vi "Get Label Settings for RT.vi"(8 "error in":errorcluster, 11 "label ref in":T1 format="%.0x") -> (0 "error out":errorcluster, 2 "label settings for RT":T2 {"Label Timestamp Channel Data Reference" format="%.0x"; "Word Initial Raw Value" format="%032.0f"; "Label Disable/Trigger Channel Reference" format="%.0x"; "parameter driver data"."Tx parameter refs" format="%.0x"; "SDI" format="%02b"; "label" format="%.0o"}, 3 "label ref out":T1 format="%.0x")   [LabVIEW 2024]
uses:
  RT Label Settings.ctl
  Label.ctl
  RT Parameters.ctl
  Parameter Definition.ctl
  <vilib>/NI/NI VeriStand Encoding and Decoding/Encoding.ctl
  <vilib>/NI VeriStand/Custom Device API/Custom Device Item Ref.ctl
  Transfer Type.ctl
  <vilib>/NI VeriStand/Custom Device API/Data Reference.ctl
  Scripting/AIM/Constants.vi
  <vilib>/NI VeriStand/Custom Device API/Get Item Property (String).vi
  <vilib>/NI VeriStand/Custom Device API/Custom Device API.lvlib
  Scripting/AIM/AIM ARINC 429 Scripting.lvlib
  <vilib>/NI/NI VeriStand Encoding and Decoding/Encoding and Decoding.lvlib
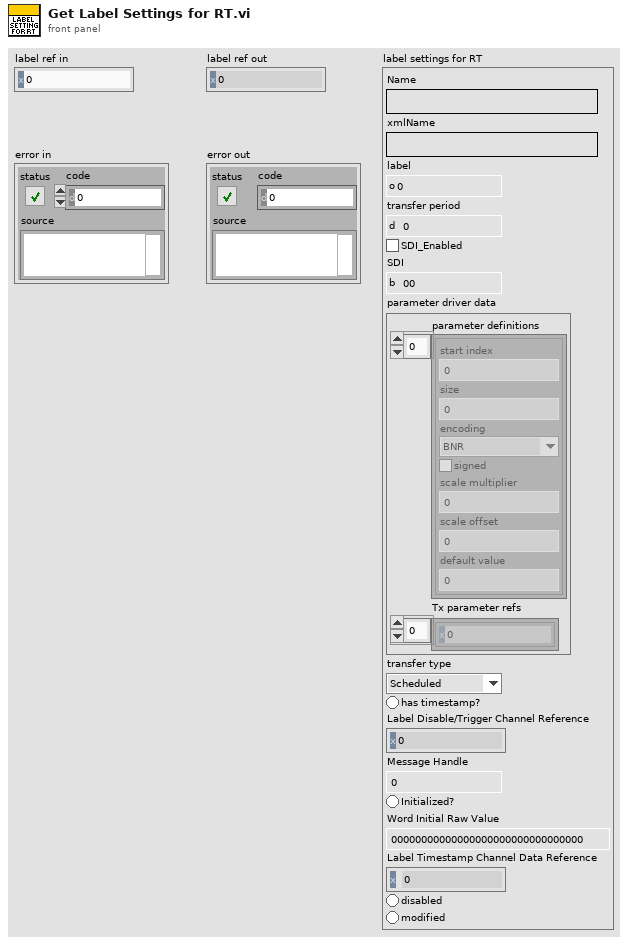
[diagram p1: front panel]
types:
  T1 = typedef "Custom Device API.lvlib/Custom Device Item Ref.ctl" = u64
  T2 = typedef "RT Label Settings.ctl" = cluster{"Name":string, "xmlName":string, "label":T3, "transfer period":u32, "SDI_Enabled":bool, "SDI":u8, "parameter driver data":T4, "transfer type":T7, "has timestamp?":bool, "Label Disable/Trigger Channel Reference":T1, "Message Handle":u64, "Initialized?":bool, "Word Initial Raw Value":u32, "Label Timestamp Channel Data Reference":T8, "disabled":bool, "modified":bool}
  T3 = typedef "Label.ctl" = u8
  T4 = typedef "RT Parameters.ctl" = cluster{"parameter definitions":T5[], "Tx parameter refs":T1[]}
  T5 = typedef "Parameter Definition.ctl" = cluster{"start index":i32, "size":i32, "encoding":T6, "signed":bool, "scale multiplier":dbl, "scale offset":dbl, "default value":dbl}
  T6 = typedef "Encoding and Decoding.lvlib/Encoding.ctl" = enum16{"BNR", "BCD", "Discrete"}
  T7 = typedef "Transfer Type.ctl" = enum16{"Scheduled", "Acyclic", "Block", "Strobe"}
  T8 = typedef "Custom Device API.lvlib/Data Reference.ctl" = i32
  T9 = typedef "Label Properties.ctl" = cluster{"label (Dec)":T3, "SDI value":u8, "SDI enabled":bool}
  T10 = typedef "Custom Device API.lvlib/Custom Device Item Info.ctl" = cluster{"Name":string, "Is Channel":bool, "GUID":string, "Is Waveform":bool}
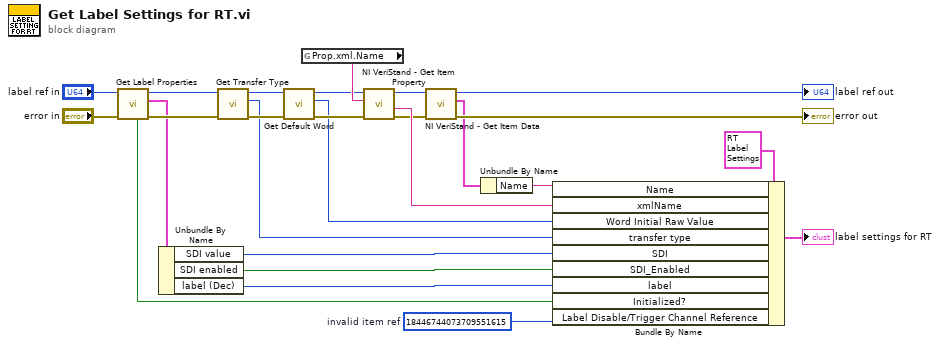
[diagram p0: block diagram]
diagram:
  w16 = T1 18446744073709551615  # invalid item ref
  n1 = call "Get Label Properties.vi"("error in"="error in", "label ref"="label ref in") -> ("error out"=w8:errorcluster, "label properties"=w4:T9, "label ref out"=w10:T1, "found?"=w5:bool)  [unwired: 6 in]
  n2 = Unbundle By Name(w4) -> ("SDI value"=w1:u8, "SDI enabled"=w2:bool, "label (Dec)"=w3:T3)
  n3 = call "Get Transfer Type.vi"("error in"=w8, "label ref"=w10) -> ("error out"=w7:errorcluster, "transfer type"=w6:T7, "label ref out"=w9:T1)  [unwired: 7 in]
  n4 = call "Get Default Word.vi"("error in"=w7, "label ref"=w9) -> ("error out"=w14:errorcluster, "default word"=w13:u32, "label ref out"=w15:T1)  [unwired: 7 in]
  n5 = global read "Constants.vi" "Prop.xml.Name"() -> (w18:string)
  n6 = call-poly <vilib>:"NI VeriStand - Get Item Property.vi"("error in (no error)"=w14, "Property Name"=w18, "Item Ref in"=w15) -> ("error out"=w20:errorcluster, "Value"=w23:string, "Item Ref out"=w19:T1)  [unwired: 5 in, 1 out]
  n7 = call <vilib>:"NI VeriStand - Get Item Data.vi"("error in (no error)"=w20, "Item Ref in"=w19) -> ("error out"=→"error out":errorcluster, "Item Info"=w17:T10, "Item Ref out"=→"label ref out":T1)  [unwired: 6 in, 1 out]
  n8 = Unbundle By Name(w17) -> ("Name"=w22:string)
  n9 = Bundle By Name(cluster=T2 {"Name"="", "xmlName"="", "label"=0, "transfer period"=0, "SDI_Enabled"=FALSE, "SDI"=0, "parameter driver data"={"parameter definitions"=[], "Tx parameter refs"=[]}, "transfer type"=enum."Scheduled", "has timestamp?"=FALSE, "Label Disable/Trigger Channel Reference"=0, "Message Handle"=0, "Initialized?"=FALSE, "Word Initial Raw Value"=0, "Label Timestamp Channel Data Reference"=0, "disabled"=FALSE, "modified"=FALSE} ("label settings for RT"), "Name"=w22, "xmlName"=w23, "Word Initial Raw Value"=w13, "transfer type"=w6, "SDI"=w1, "SDI_Enabled"=w2, "label"=w3, "Initialized?"=w5, "Label Disable/Trigger Channel Reference"=w16) -> (→"label settings for RT":T2)
